vi "3motor.vi"(8 "error in (no error)":errorcluster, 9 "Reset":bool, 10 "dt(s)":dbl, 11 "Motor speed":dbl[](array[numeric])) -> (0 "error out":errorcluster, 1 "encoder array":dbl[](array[numeric]))   [LabVIEW 2019]
uses:
  FPGA_subVIs/low level/motor/motor enum.ctl
  FPGA_subVIs/low level/motor/motor.lvlib
panel:
  out "Waveform Chart 2":T1(graph)
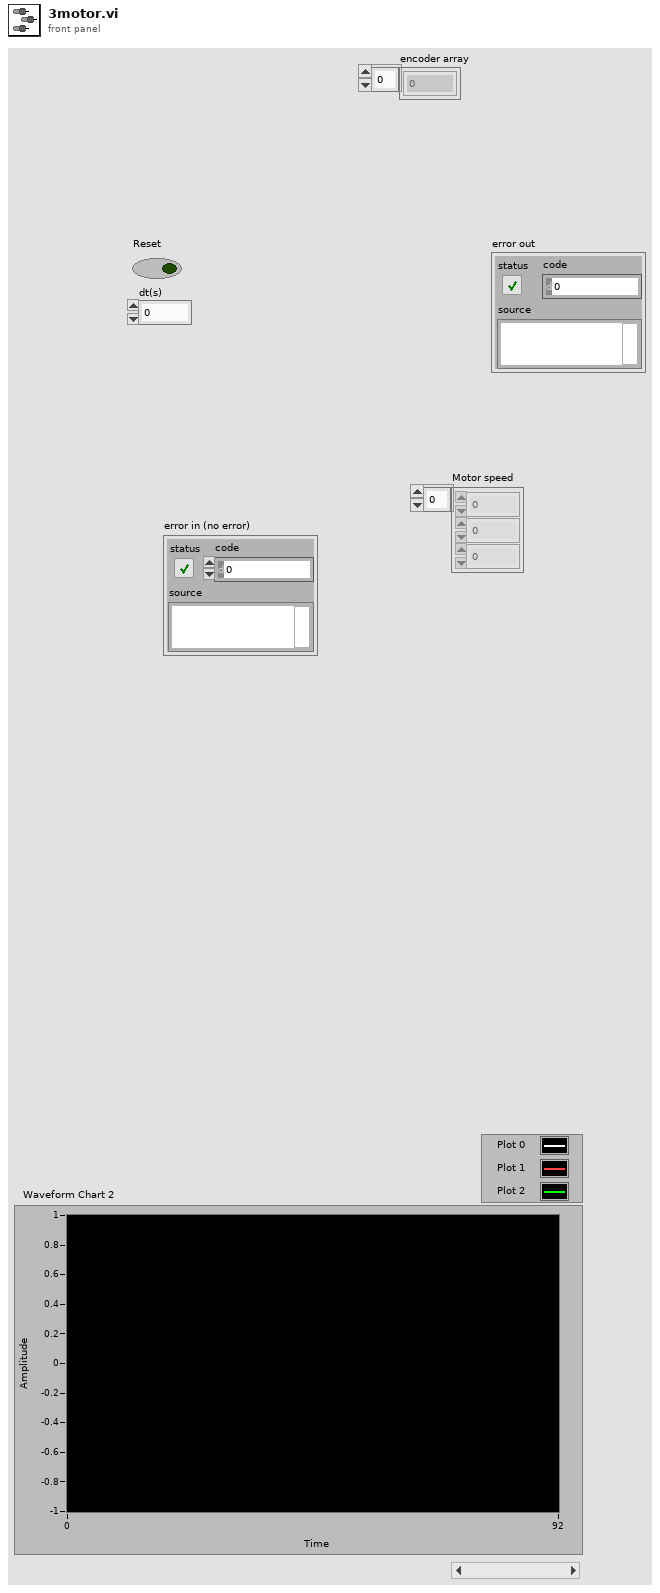
[diagram p1: front panel]
types:
  T1 = cluster{"process":dbl, "process":dbl, "process":dbl}
  T2 = typedef "my FPGA lib.lvlib/motor.lvlib/motor enum.ctl" = enum16{"M1", "M2", "M3", "M4"}
  T3 = cluster{"proportional gain (Kc)":dbl, "integral time (Ti, min)":dbl, "derivative time (Td, min)":dbl}
  T4 = cluster{"Numeric":dbl, "Numeric":dbl, "Numeric":dbl}
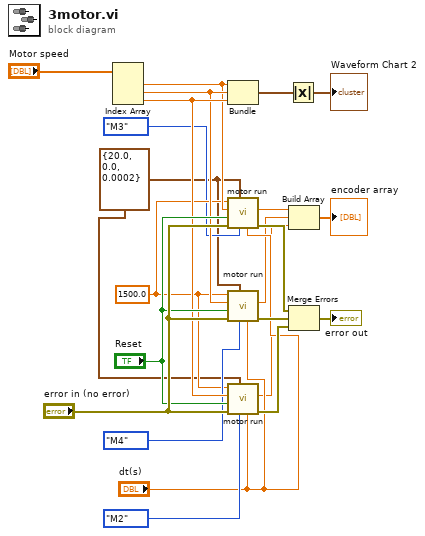
[diagram p0: block diagram]
diagram:
  w7 = 1500.0 ("PWM frequence")
  w5 = T3 {"proportional gain (Kc)"=20.0, "integral time (Ti, min)"=0.0, "derivative time (Td, min)"=0.0002} ("PID gains")
  n1 = Index Array(array="Motor speed") -> (element #1=w8:dbl, element #2=w10:dbl, element #3=w13:dbl)  [unwired: 3 in]
  n2 = Bundle("Numeric"=w8, "Numeric"=w10, "Numeric"=w13) -> (w14:T4)  [unwired: 1 in]
  n3 = call "motor run.vi"("dt(s)"="dt(s)", "motor select"=motor_enum."M3", "PID gains"=w5, "error in"="error in (no error)", "Reset"="Reset", "speed RPM"=w8, "PWM frequence"=w7) -> ("error out"=w18:errorcluster, "encoder"=w4:dbl)  [unwired: 1 in, 2 out]
  n4 = call "motor run.vi"("dt(s)"="dt(s)", "motor select"=motor_enum."M4", "PID gains"=w5, "error in"="error in (no error)", "Reset"="Reset", "speed RPM"=w10, "PWM frequence"=w7) -> ("error out"=w19:errorcluster, "encoder"=w3:dbl)  [unwired: 1 in, 2 out]
  n5 = call "motor run.vi"("dt(s)"="dt(s)", "motor select"=motor_enum."M2", "PID gains"=w5, "error in"="error in (no error)", "Reset"="Reset", "speed RPM"=w13, "PWM frequence"=w7) -> ("error out"=w20:errorcluster, "encoder"=w2:dbl)  [unwired: 1 in, 2 out]
  n6 = Absolute Value(x=w14) -> (abs(x)=→"Waveform Chart 2":T4)
  n7 = Build Array(w4, w3, w2) -> (→"encoder array":dbl[])
  n8 = Merge Errors(w18, w19, w20) -> (→"error out":errorcluster)
